vi "Keener.vi"(8 "Bottom Limit":bool, 10 "Value":dbl, 11 "Top Limit":bool) -> (3 "Output":dbl)   [LabVIEW 2014]
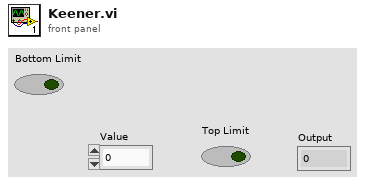
[diagram p1: front panel]
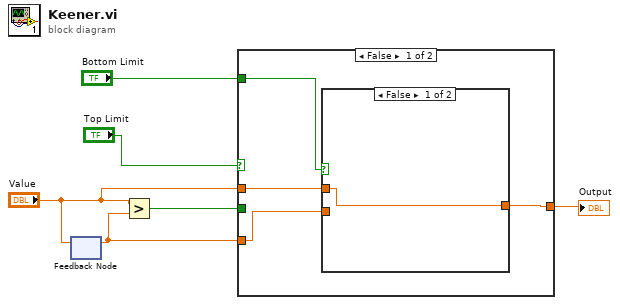
[diagram p0: block diagram]
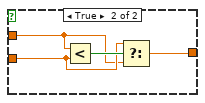
[diagram p2: hidden frame]
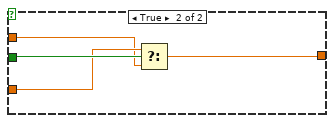
[diagram p3: hidden frame]
diagram:
  n1 = feedback-in #1("Value") -> ()
  n2 = feedback #1() -> (w4:dbl)  [unwired: 1 in]
  n3 = Greater?(x="Value", y=w4) -> (0:w5:bool)
  n4 = case shown="False" "Top Limit" {
    tunnel: w5 -> [_ w19]
    tunnel: "Value" -> [w10 w16]
    tunnel: w4 -> [w9 w17]
    tunnel: [w7 w18] -> w3
    tunnel: "Bottom Limit" -> [w8 _]
    frame False {
      n5 = case shown="False" w8 {
        tunnel: w10 -> [w11 w13]
        tunnel: w9 -> [_ w14]
        tunnel: [w11 w12] -> w7
        frame False {
        }
        frame True {
          n6 = Less?(x=w13, y=w14) -> (x < y?=w15:bool)
          n7 = Select(t=w14, s=w15, f=w13) -> (s? t:f=w12:dbl)
        }
      }
    }
    frame True {
      n8 = Select(t=w17, s=w19, f=w16) -> (s? t:f=w18:dbl)
    }
  }
  "Output" <- w3
